vi "bluetoothDiscovery.vi"() -> ()   [LabVIEW 2024]
panel:
  out "service list":T1(array[cluster])
  out "number of services":u16
  out "number of devices":u16
  in  "time limit ms (10000)":i32=10000
  out "device list":T2(array[cluster])
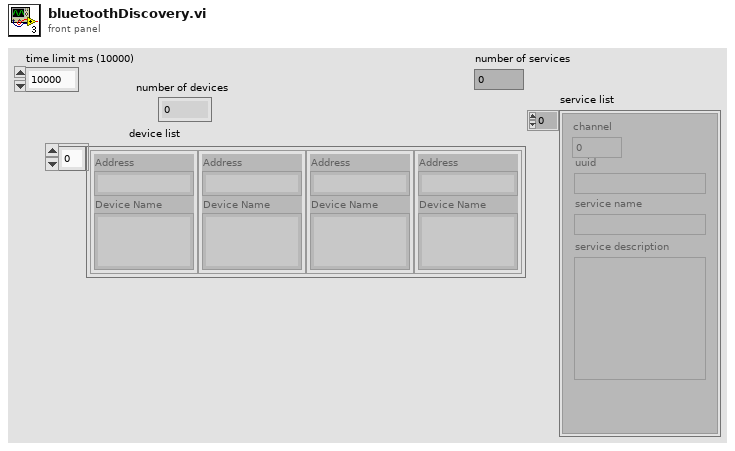
[diagram p1: front panel]
types:
  T1 = cluster{"channel":u16, "uuid":string, "service name":string, "service description":string}[]
  T2 = cluster{"Address":string, "Device Name":string}[]
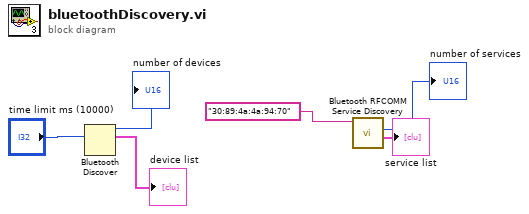
[diagram p0: block diagram]
diagram:
  n1 = Bluetooth Discover(10:"time limit ms (10000)") -> (2:→"device list":T2, 3:→"number of devices":u16)  [unwired: 1 in, 1 out]
  n2 = call <vilib>:"Bluetooth RFCOMM Service Discovery.vi"("address in"="30:89:4a:4a:94:70") -> ("service list"=→"service list":T1, "number of services"=→"number of services":u16)  [unwired: 3 in, 2 out]
